vi "CAL-Get Max SPL (waveform).vi"(0 "Cal File":path, 7 "Y":dbl[](array[numeric]), 9 "Sampling Rate (Hz)":dbl, 11 "error in (no error)":errorcluster) -> (8 "Max SPL":dbl, 15 "error out":errorcluster)   [LabVIEW 2020]
uses:
  epl-vi-lib/PXI DAQ VIs/DAQ Engine VIs/PXI Globals.vi
  epl-vi-lib/Utility VIs/Math VIs/Linear to dB (scalar).vi
  epl-vi-lib/Utility VIs/Math VIs/FFT x(t) to dB,Degrees (1D).vi
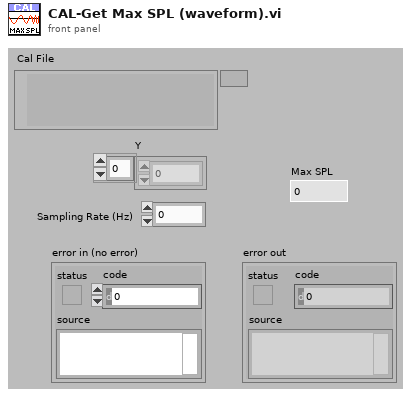
[diagram p1: front panel]
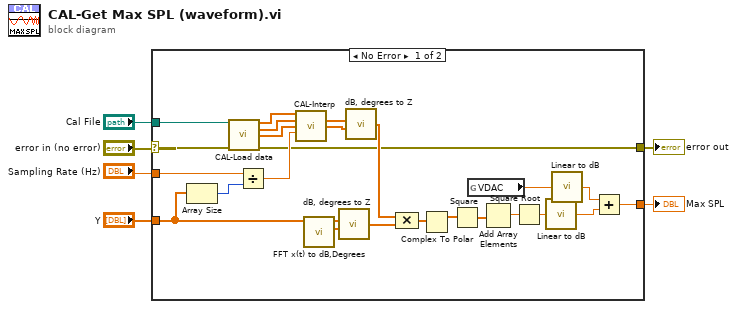
[diagram p0: block diagram]
diagram:
  n1 = case shown="No Error" "error in (no error)" {
    selector: "error in (no error)" -> [w14 w32]
    tunnel: [w13 w32] -> w5
    tunnel: "Sampling Rate (Hz)" -> [w12 _]
    tunnel: "Y" -> [w10 _]
    tunnel: [w9 _] -> w2
    tunnel: "Cal File" -> [w7 _]
    frame No Error {
      n2 = Array Size(array=w10) -> (size(s)=w11:i32)
      n3 = call "CAL-Load data.vi"("user path"=w7, "error in (no error)"=w14) -> ("Frequency (Hz)"=w27:dbl[], "Mag"=w26:dbl[], "Phase"=w25:dbl[], "error out"=w13:errorcluster)  [unwired: 6 in, 4 out]
      n4 = Divide(x=w12, y=w11) -> (x/y=w23:dbl)
      n5 = call "CAL-Interp.vi"("Frequency (Hz)"=w27, "Magnitude (dB)"=w26, "Phase (degrees)"=w25, "df (Hz)"=w23) -> ("Interp Magnitude (dB)"=w24:dbl[], "Interp Phase (degrees)"=w8:dbl[])  [unwired: 8 in, 2 out]
      n6 = call-poly "FFT x(t) to dB,Degrees.vi"("X"=w10) -> ("+Freq Phase of FFT (degrees)"=w21:dbl[], "+Freq. Mag of FFT (dB rms)"=w22:dbl[])  [unwired: 8 in, 1 out]
      n7 = call "dB, degrees to Z.vi"("Magnitude (dB)"=w22, "Phase (degrees)"=w21) -> ("Z"=w15:cdb[])  [unwired: 5 in]
      n8 = call "dB, degrees to Z.vi"("Magnitude (dB)"=w24, "Phase (degrees)"=w8) -> ("Z"=w28:cdb[])  [unwired: 5 in]
      n9 = Compound Arithmetic op=MULTIPLY(w28, w15) -> (w29:cdb[])
      n10 = Complex To Polar(r * e^(i*theta)=w29) -> (r=w17:dbl[])  [unwired: 1 out]
      n11 = Square(x=w17) -> (x^2=w20:dbl[])
      n12 = global read "PXI Globals.vi" "VDAC"() -> (w31:dbl)
      n13 = Add Array Elements(numeric array=w20) -> (sum=w19:dbl)
      n14 = Square Root(x=w19) -> (sqrt(x)=w18:dbl)
      n15 = call-poly "Linear to dB.vi"("Linear"=w18) -> ("dB"=w16:dbl)
      n16 = call-poly "Linear to dB.vi"("Linear"=w31) -> ("dB"=w30:dbl)
      n17 = Add(x=w30, y=w16) -> (x+y=w9:dbl)
    }
    frame Error {
    }
  }
  "error out" <- w5
  "Max SPL" <- w2
